vi "TemplatewError.vi"() -> ()   [LabVIEW 2017]
panel:
  in  "error in":errorcluster
  out "error out":errorcluster
  # "This is a test"
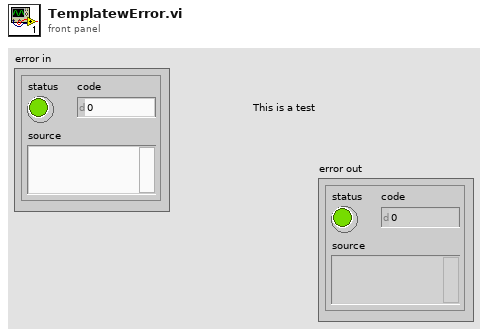
[diagram p1: front panel]
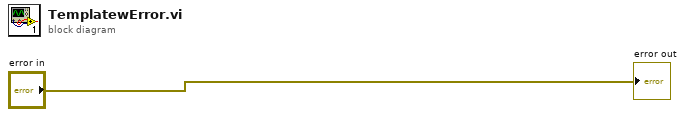
[diagram p0: block diagram]
diagram:
  "error out" <- "error in"
